vi "Variable@Select(X=A_B_C)__Parameter.vi"(1 "ParamterIn":string) -> (0 "ParamterOut":string)   [LabVIEW 2020]
panel:
  in  "Variable Section":string(combo)
  in  "C":string(combo)
  in  "B":string(combo)
  in  "Logic":string(combo)
  in  "X":string(combo)
  in  "Confirm":bool
  # "Variable@Select(X=A?B:C)"
  # "True"
  # "="
  # "False"
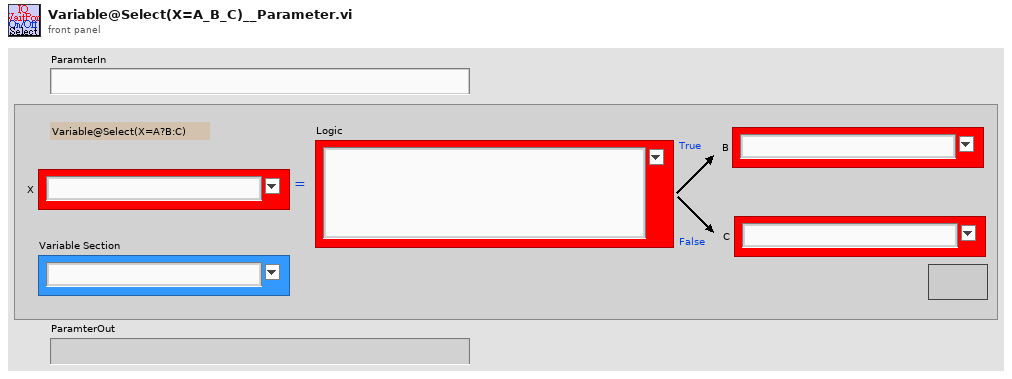
[diagram p1: front panel]
types:
  T1 = enum16{"Get", "Init", "Set", "Delete", "GetElement", "Inc", "Dec", "ReName"}
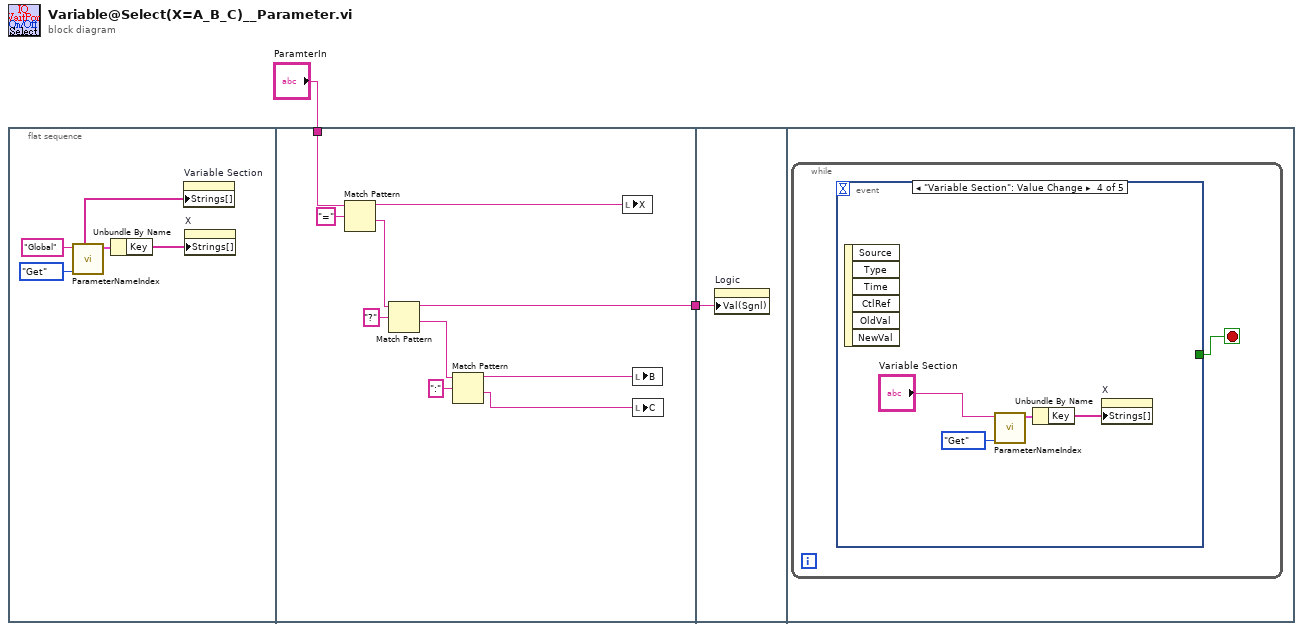
[diagram p0: block diagram]
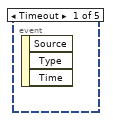
[diagram p2: hidden frame]
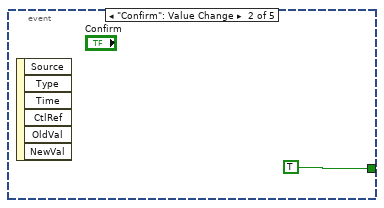
[diagram p3: hidden frame]
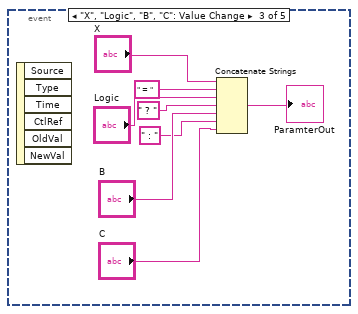
[diagram p4: hidden frame]
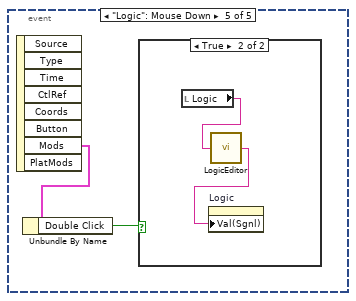
[diagram p5: hidden frame]
diagram:
  n1 = flat-sequence {
    tunnel: "ParamterIn" -> [w17]
    tunnel: [w12] -> w1
    tunnel: w1 -> [w18]
    frame #0 {
      n2 = call "ParameterNameIndex.vi"("OP"=T1."Get", "VariableSection"="Global") -> ("SectionKeyValue"=w5:cluster{"Key":string[], "Value":string[]}, "SectionList"=w3:string[])  [unwired: 3 in, 5 out]
      n3 = Unbundle By Name(w5) -> ("Key"=w4:string[])
      n4 = property on="Variable Section" class="CmbBox"("Strings[]"=w3) -> ()  [unwired: 2 in, 2 out]
      n5 = property on="X" class="CmbBox"("Strings[]"=w4) -> ()  [unwired: 2 in, 2 out]
    }
    frame #1 {
      n6 = Match Pattern(string=w17, regular expression="=") -> (before substring=w15:string, after substring=w14:string)  [unwired: 1 in, 2 out]
      n7 = Match Pattern(string=w14, regular expression="?") -> (before substring=w12:string, after substring=w11:string)  [unwired: 1 in, 2 out]
      n8 = Match Pattern(string=w11, regular expression=":") -> (before substring=w9:string, after substring=w8:string)  [unwired: 1 in, 2 out]
      n9 = local write "X"(w15) -> ()
      n10 = local write "B"(w9) -> ()
      n11 = local write "C"(w8) -> ()
    }
    frame #2 {
      n12 = property on="Logic" class="CmbBox"("Val(Sgnl)"=w18) -> ()  [unwired: 2 in, 2 out]
    }
    frame #3 {
      n13 = while {
        stop <- w19 stop-if-true
        n14 = event shown="[3] \"Variable Section\": Value Change" {
          selector: _ -> [_ _ _ _ _]
          dyn-events: _ -> [_ _ _ _ _]
          timeout: _ -> [_ _ _ _ _]
          tunnel: [_ TRUE _ _ _] -> w19
          event Timeout {
            n15 = event-data() -> ()  [unwired: 1 in, 3 out]
          }
          event "Confirm": Value Change {
            n16 = event-data() -> ()  [unwired: 1 in, 6 out]
          }
          event "X", "Logic", "B", "C": Value Change {
            n17 = event-data() -> ()  [unwired: 1 in, 6 out]
            n18 = Concatenate Strings("X", " = " ("string"), "Logic", " ? " ("string"), "B", " : " ("string"), "C") -> (→"ParamterOut":string)
          }
          event "Variable Section": Value Change {
            n19 = event-data() -> ()  [unwired: 1 in, 6 out]
            n20 = call "ParameterNameIndex.vi"("OP"=T1."Get", "VariableSection"="Variable Section") -> ("SectionKeyValue"=w32:cluster{"Key":string[], "Value":string[]})  [unwired: 3 in, 6 out]
            n21 = Unbundle By Name(w32) -> ("Key"=w29:string[])
            n22 = property on="X" class="CmbBox"("Strings[]"=w29) -> ()  [unwired: 2 in, 2 out]
          }
          event "Logic": Mouse Down {
            n23 = event-data() -> ("Mods"=w34:cluster{"Double Click":bool, "Menu Key":bool})  [unwired: 1 in, 7 out]
            n24 = Unbundle By Name(w34) -> ("Double Click"=w33:bool)
            n25 = case shown="True" w33 {
              frame False {
              }
              frame True {
                n26 = local read "Logic"() -> (w36:string)
                n27 = call "LogicEditor.vi"("Logic Express"=w36) -> ("LogicExpressOut"=w35:string)
                n28 = property on="Logic" class="CmbBox"("Val(Sgnl)"=w35) -> ()  [unwired: 2 in, 2 out]
              }
            }
          }
        }
      }
    }
  }
